vi "Update Methods Events.vi"(8 "error in (no error)":errorcluster, 11 "LVClassLibrary in":refnum<vi>) -> (0 "error out":errorcluster, 3 "LVClassLibrary out":refnum<vi>)   [LabVIEW 2019, in "gRPC Scripting Tools.lvlib"]
uses:
  gRPC Scripting Tools.lvlib
  <vilib>/event_ctls.llb/lveventtype.ctl
  TypeDefs/RPC Method Parameters.ctl
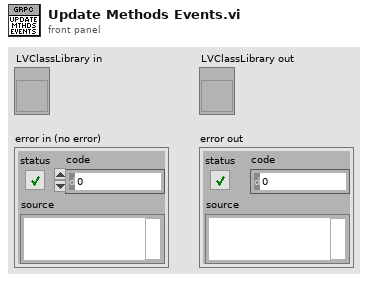
[diagram p1: front panel]
types:
  T1 = typedef "lveventtype.ctl" = enum32{"Null", "Timeout", "Annotation Menu Selection", "Annotation Menu Selection?", "App Instance Close", "App Instance Close?", "Autoscale Range Change", "Bookmark Info Change", "Cell Edit", "Cell Edit?", "Cursor Grab", "Cursor Grab?", "Cursor Menu Selection", "Cursor Menu Selection?", "Cursor Move", "Cursor Release", "Data Change", "Direction Change", "Display State Change", "Drag Ended", "Drag Enter", "Drag Leave", "Drag Over", "Drag Source Update", "Drag Starting", "Drag Starting?", "Drop", "Exec State Change", "Key Down", "Key Down?", "Key Repeat", "Key Repeat?", "Key Up", "Listbox Double Click", "Menu Activation?", "Menu Selection (App)", "Menu Selection? (App)", "Menu Selection (User)", "Mouse Down", "Mouse Down?", "Mouse Enter", "Mouse Leave", "Mouse Move", "Mouse Up", "Mouse Wheel", "NI Security User Change (App)", "Pane Size", "Panel Close", "Panel Close?", "Panel Resize", "Plot Attribute Change", "Scale Range Change", "Shortcut Menu Activation?", "Shortcut Menu Selection (App)", "Shortcut Menu Selection? (App)", "Shortcut Menu Selection (User)", "Tree Double Click", "Tree Drag", "Tree Drag?", "Tree Drop", "Tree Drop?", "Tree Item Close", "Tree Item Close?", "Tree Item Open", "Tree Item Open?", "User Event", "Value Change"}
  T2 = cluster{"Event Type":T1, "Event Registration Index":i32}[]
  T3 = typedef "gRPC Scripting Tools.lvlib/RPC Method Parameters.ctl" = cluster{"RPC Method Name":string, "Request Metadata Name":string, "Response Metadata Name":string}
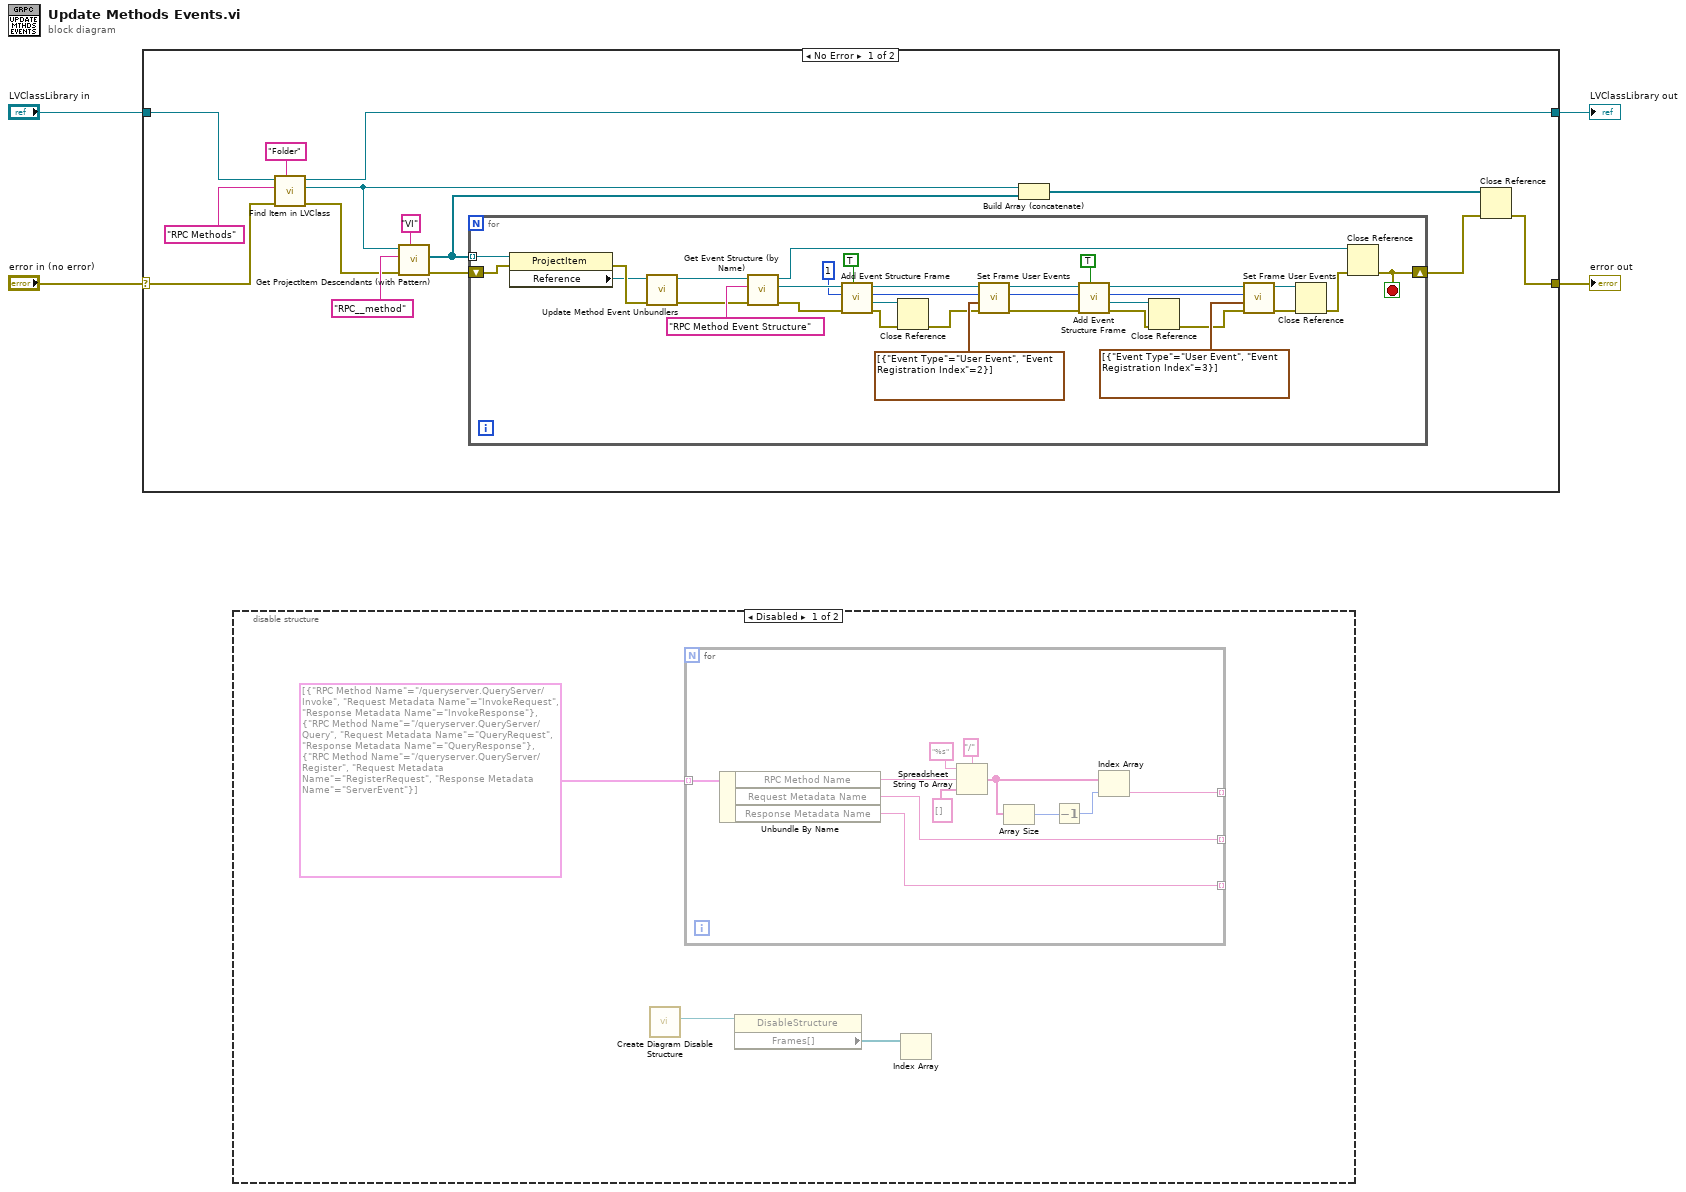
[diagram p0: block diagram]
diagram:
  n1 = case shown="No Error" "error in (no error)" {
    selector: "error in (no error)" -> [w5 w52]
    tunnel: [w17 w51] -> w4
    tunnel: "LVClassLibrary in" -> [w16 w51]
    tunnel: [w9 w52] -> w2
    frame No Error {
      n2 = call "Find Item in LVClass.vi"("Item Type"="Folder", "error in (no error)"=w5, "Item Name"="RPC Methods", "Class Item in"=w16) -> ("error out"=w12:errorcluster, "Project Item (Class Item)"=w7:refnum<vi>, "Class Item out"=w17:refnum<vi>)  [unwired: 4 in, 1 out]
      n3 = call "Get ProjectItem Descendants (with Pattern).vi"("Type"="VI", "error in (no error)"=w12, "Pattern"="RPC__method" ("regular expression"), "ProjectItem in"=w7) -> ("error out"=w11:errorcluster, "ProjectItem descendents"=w8:refnum<vi>[])  [unwired: 5 in, 1 out]
      n4 = for {
        tunnel: w8 -> [w50] mode=indexing
        shift-right: [w24] -> w10
        shift-left: w11 -> [w49]
        stop <- w24 stop-if-true
        n5 = property class="ProjectItem"(reference=w50, error in=w49) -> (error out=w48:errorcluster, "Reference"=w21:refnum<vi>)  [unwired: 1 out]
        n6 = call "Update Method Event Unbundlers.vi"("error in (no error)"=w48, "VI ref in"=w21) -> ("error out"=w45:errorcluster, "VI ref out"=w47:refnum<vi>)  [unwired: 7 in, 1 out]
        n7 = call "Get Event Structure (by Name).vi"("error in (no error)"=w45, "Label"="RPC Method Event Structure", "Owner VI in"=w47) -> ("error out"=w43:errorcluster, "Event Structure ref out"=w44:refnum<vi>, "Owner VI out"=w25:refnum<vi>)  [unwired: 5 in, 1 out]
        n8 = call "Add Event Structure Frame.vi"("After? (T)"=TRUE, "error in (no error)"=w43, "Reference Frame Index"=u32 1, "Event Structure ref in"=w44) -> ("error out"=w19:errorcluster, "Added Frame"=w20:refnum<vi>, "Added Frame Index"=w39:i32, "Event Structure ref out"=w42:refnum<vi>)  [unwired: 4 in]
        n9 = Close Reference(reference=w20, error in (no error)=w19) -> (error out=w28:errorcluster)
        n10 = call "Set Frame User Events.vi"("error in (no error)"=w28, "Dynamic Events"=T2 [{"Event Type"=enum."User Event", "Event Registration Index"=2}], "Frame Index in"=w39, "Event Structure ref in"=w42) -> ("error out"=w34:errorcluster, "Frame Index out"=w32:i32, "Event Structure ref out"=w33:refnum<vi>)  [unwired: 5 in]
        n11 = call "Add Event Structure Frame.vi"("After? (T)"=TRUE, "error in (no error)"=w34, "Reference Frame Index"=w32, "Event Structure ref in"=w33) -> ("error out"=w22:errorcluster, "Added Frame"=w23:refnum<vi>, "Added Frame Index"=w36:i32, "Event Structure ref out"=w35:refnum<vi>)  [unwired: 4 in]
        n12 = Close Reference(reference=w23, error in (no error)=w22) -> (error out=w27:errorcluster)
        n13 = call "Set Frame User Events.vi"("error in (no error)"=w27, "Dynamic Events"=T2 [{"Event Type"=enum."User Event", "Event Registration Index"=3}], "Frame Index in"=w36, "Event Structure ref in"=w35) -> ("error out"=w30:errorcluster, "Event Structure ref out"=w29:refnum<vi>)  [unwired: 5 in, 1 out]
        n14 = Close Reference(reference=w29, error in (no error)=w30) -> (error out=w26:errorcluster)
        n15 = Close Reference(reference=w25, error in (no error)=w26) -> (error out=w24:errorcluster)
      }
      n16 = Build Array (concatenate)(w7, w8) -> (w6:refnum<vi>[])
      n17 = Close Reference(reference=w6, error in (no error)=w10) -> (error out=w9:errorcluster)
    }
    frame Error {
    }
  }
  "error out" <- w2
  "LVClassLibrary out" <- w4
  n18 = disable-structure shown="Disabled" {
    frame Disabled {
      n19 = call "Create Diagram Disable Structure.vi"() -> ("DDS  Ref out"=w53:refnum<vi>)  [unwired: 9 in, 2 out]
      n20 = for {
        tunnel: T3[] [{"RPC Method Name"="/queryserver.QueryServer/Invoke", "Request Metadata Name"="InvokeRequest", "Response Metadata Name"="InvokeResponse"}, {"RPC Method Name"="/queryserver.QueryServer/Query", "Request Metadata Name"="QueryRequest", "Response Metadata Name"="QueryResponse"}, {"RPC Method Name"="/queryserver.QueryServer/Register", "Request Metadata Name"="RegisterRequest", "Response Metadata Name"="ServerEvent"}] ("RPC Method Parameters") -> [w66] mode=indexing
        tunnel: [w58] -> _ mode=indexing
        tunnel: [w57] -> _ mode=indexing
        tunnel: [w56] -> _ mode=indexing
        n21 = Unbundle By Name(w66) -> ("RPC Method Name"=w59:string, "Request Metadata Name"=w57:string, "Response Metadata Name"=w56:string)
        n22 = Spreadsheet String To Array(delimiter (Tab)="/", format string="%s", spreadsheet string=w59, array type (2D Dbl)=string[] []) -> (array=w60:string[])
        n23 = Array Size(array=w60) -> (size(s)=w62:i32)
        n24 = Decrement(x=w62) -> (x-1=w61:i32)
        n25 = Index Array(array=w60, index=w61) -> (element=w58:string)
      }
      n26 = property class="DisableStructure"(reference=w53) -> ("Frames[]"=w54:refnum<vi>[])  [unwired: 1 in, 2 out]
      n27 = Index Array(array=w54) -> ()  [unwired: 1 in, 1 out]
    }
    frame Enabled {
    }
  }
